vi "niDTS WLAN DSSS Tx Test UTIL DSSS ModAcc Settings to WLAN ModAcc Settings.vi"(10 "DSSS ModAcc Measurement Paramaters":T3={"ModAcc Enable"=FALSE, "Header Detection"=enum."MANUAL", "Averages"=0, "CFO Estimation"=enum."PAMBLE", "DC Offset Compensation"=FALSE, "Chip Start Location"=0, "Max Chips Used"=16, "Pulse Shaping FilterType"=enum."GAUSSIAN", "Pulse Shaping Filter Coefficient"=0.35, "Equalization"=TRUE, "Phase Tracking"=TRUE}) -> (1 "DSSS ModAcc Measurement Parameters":T1={"DC Offset Compensation"=TRUE, "Equalization"=TRUE, "Phase Tracking"=TRUE, "Chip Start Location"=0, "Max Chips Used"=16, "Pulse Shaping FilterType"=enum."GAUSSIAN", "Pulse Shaping Filter Coefficient"=0.35}, 2 "ModAcc Measurement Paramaters":T4={"ModAcc Enable"=FALSE, "Header Detection"=enum."MANUAL", "Averages"=3, "Amplitude Tracking"=FALSE, "Channel Tracking"=FALSE, "Time Tracking"=TRUE, "Phase Tracking"=enum."NONE", "Clock Offset Est"=FALSE, "Impairments Est"=FALSE, "CFO Estimation"=enum."PAMBLE"})   [LabVIEW 2014, in "niDTS WLAN.lvlib"]
uses:
  niDTS WLAN.lvlib
  Includes/niDTS WLAN INC ModAcc Measurement Parameters.ctl
  Includes/niDTS WLAN DSSS Tx Test INC ModAcc Measurement Parameters.ctl
  Includes/niDTS WLAN INC Pulse Shaping Filter Type.ctl
  Includes/niDTS WLAN INC DSSS ModAcc Measurement Parameters.ctl
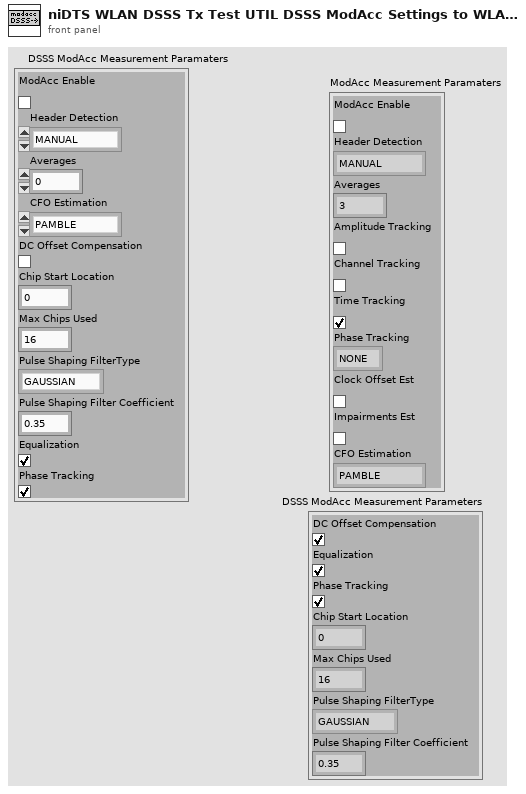
[diagram p1: front panel]
types:
  T1 = typedef "niDTS WLAN.lvlib/niDTS WLAN INC DSSS ModAcc Measurement Parameters.ctl" = cluster{"DC Offset Compensation":bool, "Equalization":bool, "Phase Tracking":bool, "Chip Start Location":i16, "Max Chips Used":i16, "Pulse Shaping FilterType":T2, "Pulse Shaping Filter Coefficient":dbl}
  T2 = typedef "niDTS WLAN.lvlib/niDTS WLAN INC Pulse Shaping Filter Type.ctl" = enum16{"NONE", "RCOSINE", "RRCOSINE", "GAUSSIAN"}
  T3 = typedef "niDTS WLAN.lvlib/niDTS WLAN DSSS Tx Test INC ModAcc Measurement Parameters.ctl" = cluster{"ModAcc Enable":bool, "Header Detection":enum16{"MANUAL", "FIRST", "ALL"}, "Averages":i32, "CFO Estimation":enum16{"PAMBLE", "PDATA"}, "DC Offset Compensation":bool, "Chip Start Location":i16, "Max Chips Used":i16, "Pulse Shaping FilterType":T2, "Pulse Shaping Filter Coefficient":dbl, "Equalization":bool, "Phase Tracking":bool}
  T4 = typedef "niDTS WLAN.lvlib/niDTS WLAN INC ModAcc Measurement Parameters.ctl" = cluster{"ModAcc Enable":bool, "Header Detection":enum16{"MANUAL", "FIRST", "ALL"}, "Averages":i32, "Amplitude Tracking":bool, "Channel Tracking":bool, "Time Tracking":bool, "Phase Tracking":enum16{"NONE", "STANDARD", "CSF", "INSTANT"}, "Clock Offset Est":bool, "Impairments Est":bool, "CFO Estimation":enum16{"PAMBLE", "PDATA"}}
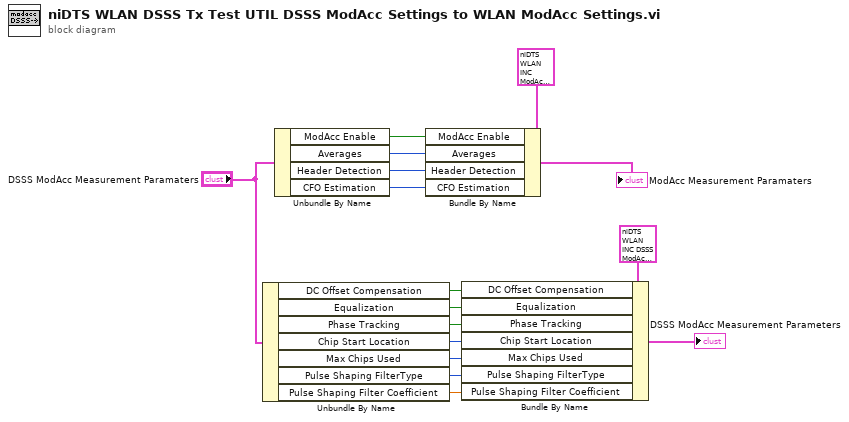
[diagram p0: block diagram]
diagram:
  n1 = Unbundle By Name("DSSS ModAcc Measurement Paramaters") -> ("DC Offset Compensation"=w8:bool, "Equalization"=w7:bool, "Phase Tracking"=w6:bool, "Chip Start Location"=w5:i16, "Max Chips Used"=w4:i16, "Pulse Shaping FilterType"=w3:T2, "Pulse Shaping Filter Coefficient"=w2:dbl)
  n2 = Unbundle By Name("DSSS ModAcc Measurement Paramaters") -> ("ModAcc Enable"=w11:bool, "Averages"=w15:i32, "Header Detection"=w14:enum16{"MANUAL", "FIRST", "ALL"}, "CFO Estimation"=w13:enum16{"PAMBLE", "PDATA"})
  n3 = Bundle By Name(cluster=T4 {"ModAcc Enable"=FALSE, "Header Detection"=enum."MANUAL", "Averages"=3, "Amplitude Tracking"=FALSE, "Channel Tracking"=FALSE, "Time Tracking"=TRUE, "Phase Tracking"=enum."NONE", "Clock Offset Est"=FALSE, "Impairments Est"=FALSE, "CFO Estimation"=enum."PDATA"} ("ModAcc Measurement Paramaters"), "ModAcc Enable"=w11, "Averages"=w15, "Header Detection"=w14, "CFO Estimation"=w13) -> (→"ModAcc Measurement Paramaters":T4)
  n4 = Bundle By Name(cluster=T1 {"DC Offset Compensation"=TRUE, "Equalization"=TRUE, "Phase Tracking"=TRUE, "Chip Start Location"=0, "Max Chips Used"=16, "Pulse Shaping FilterType"=enum."GAUSSIAN", "Pulse Shaping Filter Coefficient"=0.35} ("ModAcc DSSS Paramaters"), "DC Offset Compensation"=w8, "Equalization"=w7, "Phase Tracking"=w6, "Chip Start Location"=w5, "Max Chips Used"=w4, "Pulse Shaping FilterType"=w3, "Pulse Shaping Filter Coefficient"=w2) -> (→"DSSS ModAcc Measurement Parameters":T1)
